vi "Sig2MS getSpectraSignal.vi"(8 "error in (no error)":errorcluster, 9 "signal in":waveform(sgl), 11 "Sig2MS in":refnum<class "Sig2MS.lvclass">) -> (0 "error out":errorcluster, 3 "Sig2MS out":refnum<class "Sig2MS.lvclass">)   [LabVIEW 2018, in "Sig2MS.lvclass"]
uses:
  Sig2MS.lvclass
  Sig2MS.lvclass/Sig2MS.ctl
  DataXML/DataXML.lvclass
  SigInfo/SigInfo.lvclass
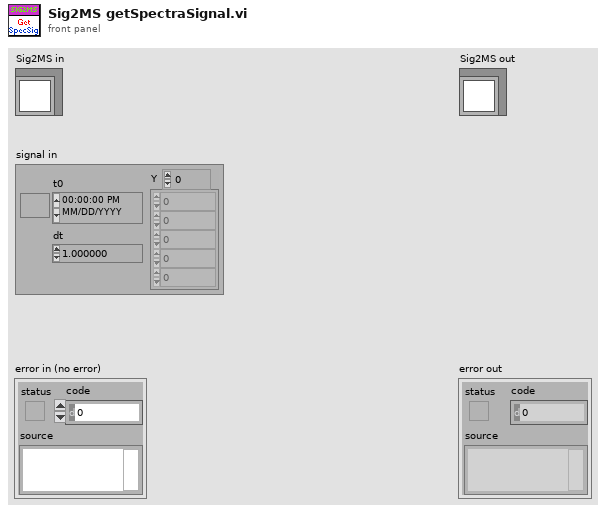
[diagram p1: front panel]
types:
  T1 = cluster{"priDt":dbl, "priXData":dbl[], "priYData":sgl[], "beta":dbl[]}[]
  T2 = cluster{"priDt":dbl, "priXData":dbl[], "priYData":sgl[], "beta":dbl[]}
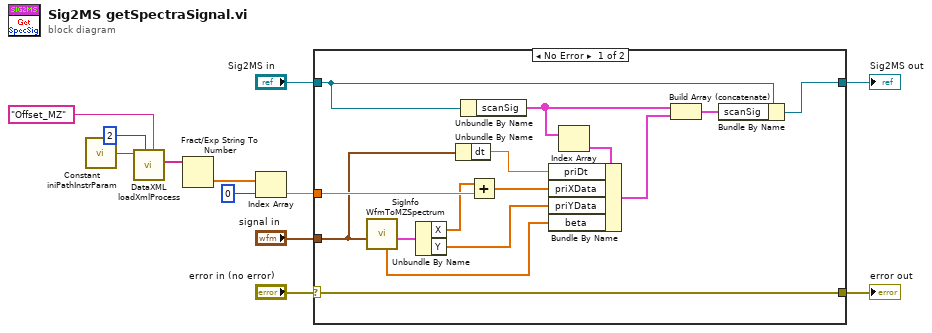
[diagram p0: block diagram]
diagram:
  n1 = call "Constant iniPathInstrParam.vi"() -> ("appended path"=w7:path)
  n2 = call "DataXML loadXmlProcess.vi"("target name"="Offset_MZ", "level"=u8 2, "xml_data_path"=w7) -> ("value"=w8:string[])  [unwired: 5 in, 3 out]
  n3 = Fract/Exp String To Number(string=w8) -> (number=w4:dbl[])  [unwired: 3 in, 1 out]
  n4 = Index Array(array=w4, index=0) -> (element=w2:dbl)
  n5 = case shown="No Error" "error in (no error)" {
    selector: "error in (no error)" -> [w27 w29]
    tunnel: [w27 w29] -> w9
    tunnel: [w26 w28] -> w12
    tunnel: "Sig2MS in" -> [w25 w28]
    tunnel: w2 -> [w22 _]
    tunnel: "signal in" -> [w21 _]
    frame No Error {
      n6 = call "SigInfo WfmToMZSpectrum.vi"("SectionalSignal"=w21) -> ("MassSpectrum"=w20:cluster{"X":dbl[], "Y":sgl[]}, "beta"=w14:dbl[])  [unwired: 8 in, 1 out]
      n7 = Unbundle By Name(w20) -> ("X"=w19:dbl[], "Y"=w15:sgl[])
      n8 = Unbundle By Name(w21) -> ("dt"=w17:dbl)
      n9 = Unbundle By Name(w25) -> ("scanSig"=w23:T1)
      n10 = Add(x=w19, y=w22) -> (x+y=w16:dbl[])
      n11 = Index Array(array=w23) -> (element=w18:T2)  [unwired: 1 in]
      n12 = Bundle By Name(cluster=w18, "priDt"=w17, "priXData"=w16, "priYData"=w15, "beta"=w14) -> (w13:T2)
      n13 = Build Array (concatenate)(w23, w13) -> (w24:T1)
      n14 = Bundle By Name(cluster=w25, "scanSig"=w24) -> (w26:refnum<class "Sig2MS.lvclass">)
    }
    frame Error {
    }
  }
  "error out" <- w9
  "Sig2MS out" <- w12
